vi "LVProjectShortcut_Item_Init.vi"(11 "Object":T1) -> ()   [LabVIEW 2017]
uses:
  <resource>/Framework/Providers/API/ItemRef.ctl
  <resource>/Framework/Providers/API/mxLvUpdateUI.ctl
  <resource>/Framework/Providers/API/mxLvChangeType.ctl
panel:
  out "error out":errorcluster
  in  "error in":errorcluster
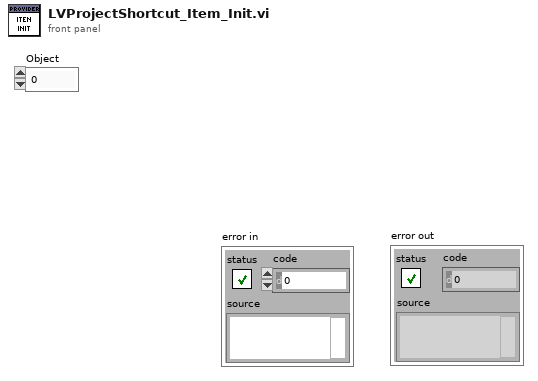
[diagram p1: front panel]
types:
  T1 = typedef "ItemRef.ctl" = u64
  T2 = typedef "mxLvChangeType.ctl" = enum32{"Item Created", "Item Modified", "File Modified", "File Deleted", "Item Added", "Item Added to SCC", "Item Renamed", "Item Modified For SCC"}
  T3 = typedef "mxLvUpdateUI.ctl" = cluster{"Action":u32, "Optional param 1":string, "Optional param 2":i32, "Optional param 3":string}
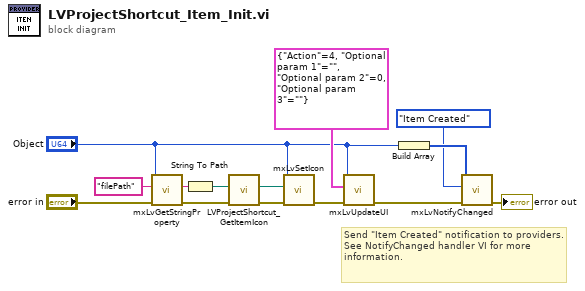
[diagram p0: block diagram]
diagram:
  # "Send \"Item Created\" notification to providers. See NotifyChanged handler VI for more information."
  n1 = call <resource>:"mxLvGetStringProperty.vi"("Error In"="error in", "Tag"="filePath", "Item"="Object") -> ("Error Out"=w11:errorcluster, "Value"=w12:string)  [unwired: 6 in, 1 out]
  n2 = String To Path(string=w12) -> (path=w10:path)
  n3 = call <resource>:"LVProjectShortcut_GetItemIcon.vi"("error in (no error)"=w11, "File Path"=w10) -> ("error out"=w8:errorcluster, "Icon Path"=w9:path)  [unwired: 8 in]
  n4 = call <resource>:"mxLvSetIcon.vi"("error in"=w8, "Icon Path"=w9, "Item"="Object") -> ("error out"=w7:errorcluster)  [unwired: 7 in, 1 out]
  n5 = call <resource>:"mxLvUpdateUI.vi"("error in"=w7, "Update UI Settings"=T3 {"Action"=4, "Optional param 1"="", "Optional param 2"=0, "Optional param 3"=""}, "Item"="Object") -> ("error out"=w5:errorcluster)  [unwired: 7 in, 1 out]
  n6 = Build Array("Object") -> (w2:T1[])
  n7 = call <resource>:"mxLvNotifyChanged.vi"("error in (no error)"=w5, "Change Type"=mxLvChangeType."Item Created", "Items"=w2) -> ("error out"=→"error out":errorcluster)  [unwired: 7 in, 1 out]
